vi "Convert Digital Output Level Units.vi"(9 "new output level units":T1, 10 "previous output level units":T1, 11 "previous output level":dbl) -> (3 "new output level":dbl)   [LabVIEW 2023]
uses:
  controls/digital output level units.ctl
  controls/audio controls.lvlib
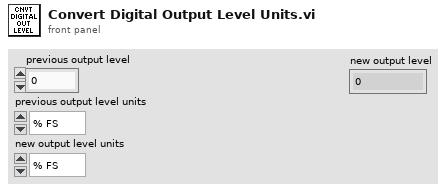
[diagram p1: front panel]
types:
  T1 = typedef "audio controls.lvlib/digital output level units.ctl" = enum32{"% FS", "dBFS", "V"}
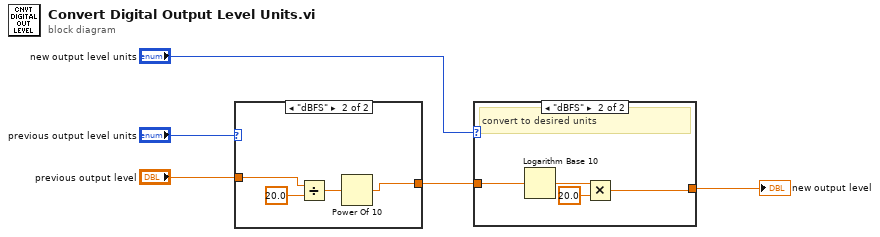
[diagram p0: block diagram]
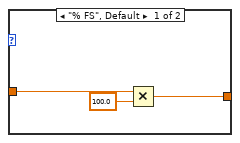
[diagram p2: hidden frame]
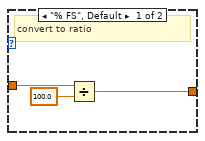
[diagram p3: hidden frame]
diagram:
  n1 = case shown="\"dBFS\"" "previous output level units" {
    tunnel: "previous output level" -> [w8 w10]
    tunnel: [w6 w9] -> w2
    frame "% FS", Default {
      # "convert to ratio"
      n2 = Divide(x=w8, y=100.0) -> (x/y=w6:dbl)
    }
    frame "dBFS" {
      n3 = Divide(x=w10, y=20.0) -> (x/y=w12:dbl)
      n4 = Power Of 10(x=w12) -> (10^x=w9:dbl)
    }
  }
  n5 = case shown="\"dBFS\"" "new output level units" {
    tunnel: w2 -> [w15 w19]
    tunnel: [w13 w17] -> w1
    frame "% FS", Default {
      n6 = Multiply(x=w15, y=100.0) -> (x*y=w13:dbl)
    }
    frame "dBFS" {
      # "convert to desired units"
      n7 = Logarithm Base 10(1:w19) -> (0:w18:dbl)
      n8 = Multiply(x=w18, y=20.0) -> (x*y=w17:dbl)
    }
  }
  "new output level" <- w1
